vi "Resistor Measure(NI9220).vi"() -> ()   [LabVIEW 2013]
uses:
  <vilib>/DAQmx/read.llb/DAQmx Read (Analog DBL 1Chan 1Samp).vi
  <vilib>/DAQmx/configure/timing.llb/DAQmx Timing (Sample Clock).vi
  <vilib>/DAQmx/create/channels.llb/DAQmx Create Channel (AI-Voltage-Basic).vi
  <vilib>/DAQmx/miscellaneous.llb/DAQmx Fill In Error Info.vi
panel:
  out "error out":errorcluster
  in  "열거형":enum16{"initial", "measure", "stop"}(ring)
  in  "error in (no error)":errorcluster caption="에러 입력(에러 없음)"
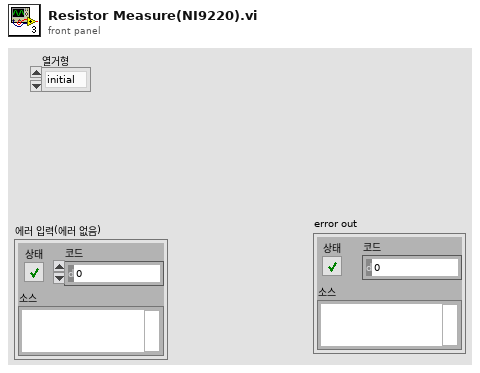
[diagram p1: front panel]
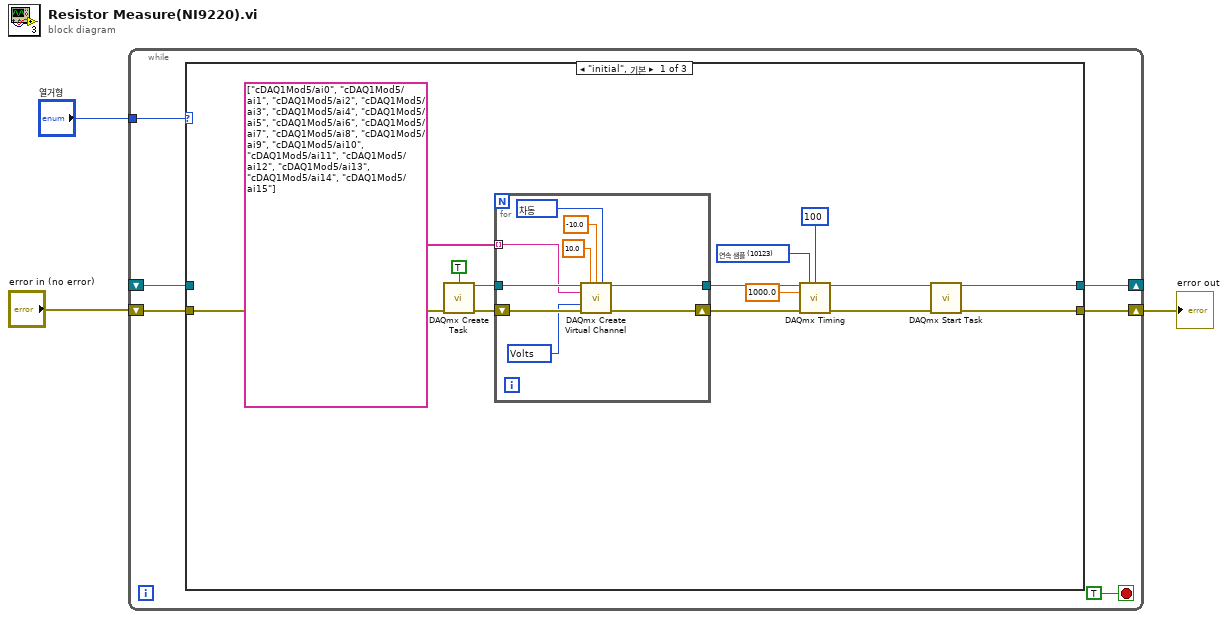
[diagram p0: block diagram]
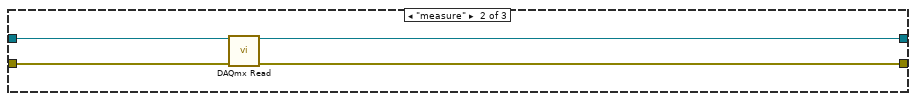
[diagram p2: hidden frame]
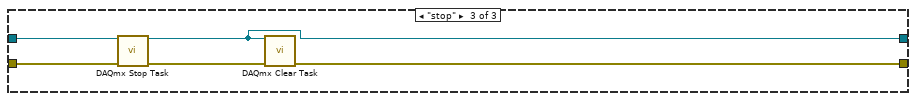
[diagram p3: hidden frame]
diagram:
  n1 = while {
    shift-right: [w6] -> w1
    shift-left: "error in (no error)" -> [w7]
    tunnel: "열거형" -> [w8]
    shift-right: [w5] -> _
    shift-left: _ -> [w4]
    stop <- TRUE stop-if-true
    n2 = case shown="\"initial\", 기본" w8 {
      tunnel: w7 -> [w19 w35 w40]
      tunnel: [w11 w33 w38] -> w6
      tunnel: [w10 w34 w37] -> w5
      tunnel: w4 -> [_ w36 w41]
      frame "initial", Default {
        w14 = 10123 items=["유한 샘플"=10178, "연속 샘플"=10123, "하드웨어 타이밍에 의한 단일 포인트"=12522] ("sample mode")
        n3 = call <vilib>:"DAQmx Create Task.vi"("auto cleanup"=TRUE, "error in"=w19) -> ("task out"=w22:refnum<k21>, "error out"=w20:errorcluster)  [unwired: 12 in]
        n4 = for {
          tunnel: w22 -> [w32]
          tunnel: tag[] ["cDAQ1Mod5/ai0", "cDAQ1Mod5/ai1", "cDAQ1Mod5/ai2", "cDAQ1Mod5/ai3", "cDAQ1Mod5/ai4", "cDAQ1Mod5/ai5", "cDAQ1Mod5/ai6", "cDAQ1Mod5/ai7", "cDAQ1Mod5/ai8", "cDAQ1Mod5/ai9", "cDAQ1Mod5/ai10", "cDAQ1Mod5/ai11", "cDAQ1Mod5/ai12", "cDAQ1Mod5/ai13", "cDAQ1Mod5/ai14", "cDAQ1Mod5/ai15"] -> [w31] mode=indexing
          tunnel: [w25] -> w18
          shift-right: [w24] -> w17
          shift-left: w20 -> [w30]
          w26 = 10106 items=["기본값"=-1, "RSE"=10083, "NRSE"=10078, "차동"=10106, "유사 차동"=12529] ("input terminal configuration")
          w29 = 10348 items=["Volts"=10348, "사용자 스케일로부터"=10065] ("units")
          n5 = call-poly <vilib>:"DAQmx Create Virtual Channel.vi"("task in"=w32, "maximum value"=10.0, "minimum value"=-10.0, "input terminal configuration"=w26, "physical channels"=w31, "units"=w29, "error in"=w30) -> ("task out"=w25:refnum<k21>, "error out"=w24:errorcluster)  [unwired: 7 in]
        }
        n6 = call-poly <vilib>:"DAQmx Timing.vi"("task/channels in"=w18, "sample mode"=w14, "samples per channel"=100, "rate"=1000.0, "error in"=w17) -> ("task out"=w13:refnum<k21>, "error out"=w12:errorcluster)  [unwired: 9 in]
        n7 = call <vilib>:"DAQmx Start Task.vi"("task/channels in"=w13, "error in"=w12) -> ("task out"=w10:refnum<k21>, "error out"=w11:errorcluster)  [unwired: 12 in]
      }
      frame "measure" {
        n8 = call-poly <vilib>:"DAQmx Read.vi"("task/channels in"=w36, "error in"=w35) -> ("task out"=w34:refnum<k21>, "error out"=w33:errorcluster)  [unwired: 11 in, 1 out]
      }
      frame "stop" {
        n9 = call <vilib>:"DAQmx Stop Task.vi"("task/channels in"=w41, "error in"=w40) -> ("task out"=w37:refnum<k21>, "error out"=w39:errorcluster)  [unwired: 12 in]
        n10 = call <vilib>:"DAQmx Clear Task.vi"("task in"=w37, "error in"=w39) -> ("error out"=w38:errorcluster)  [unwired: 13 in]
      }
    }
  }
  "error out" <- w1
